vi "GetForLoopCount.vi"(6 "error in":errorcluster, 9 "ForLoop in":refnum<class "ForLoop.lvclass">) -> (0 "error out":errorcluster, 3 "ForLoop out":refnum<class "ForLoop.lvclass">, 4 "count UID":i32)   [LabVIEW 2014, in "Raspberry Pi Compatible Compiler for LabVIEW.lvlib" / "ForLoop.lvclass"]
uses:
  ForLoop.lvclass
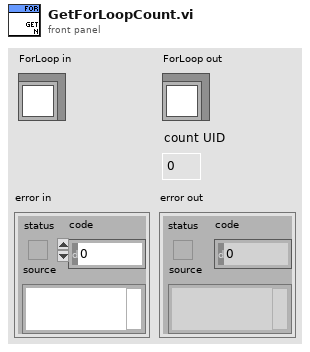
[diagram p1: front panel]
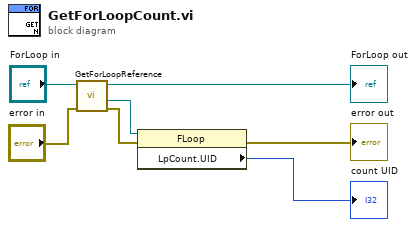
[diagram p0: block diagram]
diagram:
  n1 = call "GetForLoopReference.vi"("error in"="error in", "ForLoop in"="ForLoop in") -> ("error out"=w4:errorcluster, "reference out"=w5:refnum<vi>, "ForLoop out"=→"ForLoop out":refnum<class "ForLoop.lvclass">)  [unwired: 7 in]
  n2 = property class="FLoop"(reference=w5, error in=w4) -> (error out=→"error out":errorcluster, "LpCount.UID"=→"count UID":i32)  [unwired: 1 out]
